vi "W7X2DPut.vi"(0 "SigLabel":string, 1 "Unit":string, 5 "SigJSONbuffer":string, 7 "values":T1(array[cluster]), 8 "dimensions":i64[](array[numeric])=[1399090569999999999, -1], 9 "sample rate":u16, 11 "sample period":dbl, 12 "pulse_length":dbl) -> (2 "headers parms":string, 3 "headers":string, 4 "body":string, 6 "body Parlog":string, 10 "file path written":string, 14 "Parlog error out":errorcluster)   [LabVIEW 2014]
uses:
  <vilib>/httpClient/POSTBuffer.vi
  <vilib>/httpClient/LabVIEWHTTPClient.lvlib
panel:
  out "JSON string":string
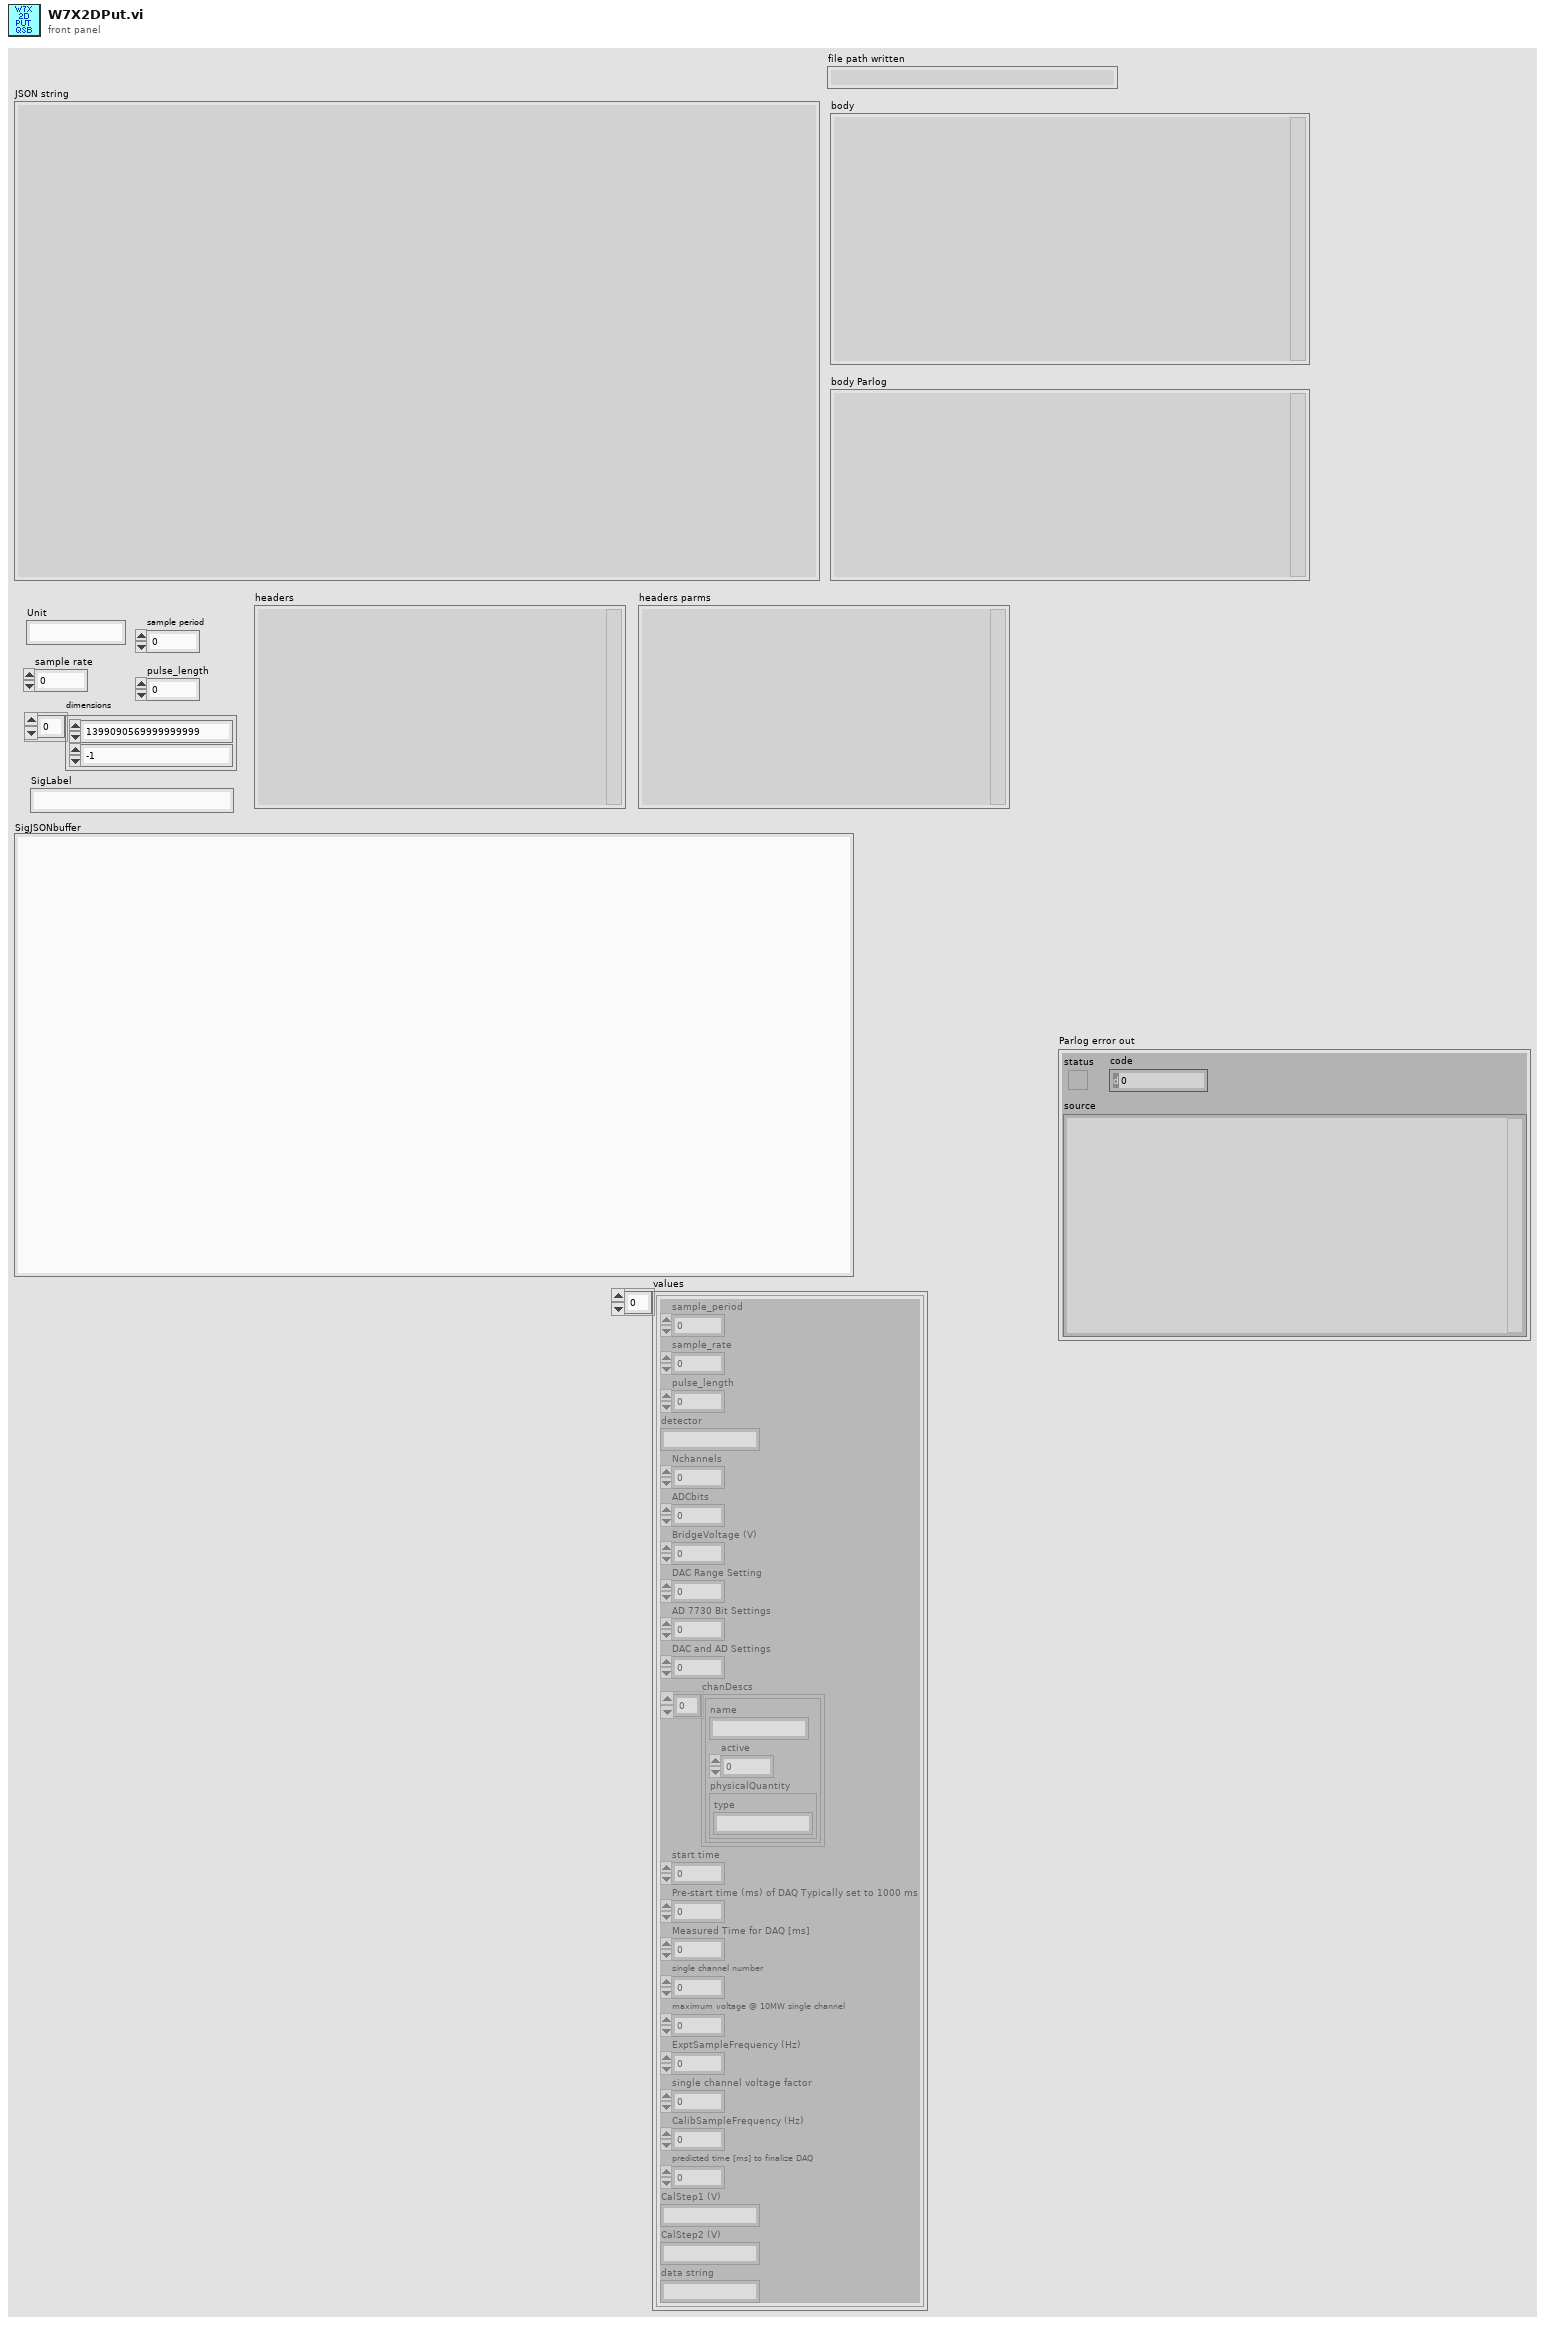
[diagram p1: front panel]
types:
  T1 = cluster{"sample_period":dbl, "sample_rate":dbl, "pulse_length":dbl, "detector":string, "Nchannels":i16, "ADCbits":i16, "BridgeVoltage (V)":sgl, "DAC Range Setting":u8, "AD 7730 Bit Settings":i32, "DAC and AD Settings":i32, "chanDescs":cluster{"name":string, "active":i32, "physicalQuantity":cluster{"type":string}}[], "start time":i64, "Pre-start time (ms) of DAQ Typically set to 1000 ms":i32, "Measured Time for DAQ [ms] ":u32, "single channel number":i64, "maximum voltage @ 10MW single channel":dbl, "ExptSampleFrequency (Hz)":sgl, "single channel voltage factor":dbl, "CalibSampleFrequency (Hz)":sgl, "predicted time [ms] to finalize DAQ":dbl, "CalStep1 (V)":string, "CalStep2 (V)":string, "data string":string}[]
  T2 = cluster{"sample_period":dbl, "sample_rate":dbl, "pulse_length":dbl, "detector":string, "Nchannels":i16, "ADCbits":i16, "BridgeVoltage (V)":sgl, "DAC Range Setting":u8, "AD 7730 Bit Settings":i32, "DAC and AD Settings":i32, "chanDescs":cluster{"name":string, "active":i32, "physicalQuantity":cluster{"type":string}}[], "start time":i64, "Pre-start time (ms) of DAQ Typically set to 1000 ms":i32, "Measured Time for DAQ [ms] ":u32, "single channel number":i64, "maximum voltage @ 10MW single channel":dbl, "ExptSampleFrequency (Hz)":sgl, "single channel voltage factor":dbl, "CalibSampleFrequency (Hz)":sgl, "predicted time [ms] to finalize DAQ":dbl, "CalStep1 (V)":string, "CalStep2 (V)":string, "data string":string}
  T3 = cluster{"name":string, "active":i32, "physicalQuantity":cluster{"type":string}}[]
  T4 = cluster{"name":string, "active":i32, "physicalQuantity":cluster{"type":string}}
  T5 = typedef "LabVIEWHTTPClient.lvlib/ClientHandle.ctl" = refnum<k1>
  T6 = cluster{"label":string, "values":cluster{"sample_period":dbl, "sample_rate":dbl, "pulse_length":dbl, "detector":string, "Nchannels":i16, "ADCbits":i16, "BridgeVoltage (V)":sgl, "DAC Range Setting":u8, "AD 7730 Bit Settings":i32, "DAC and AD Settings":i32, "chanDescs":cluster{"name":string, "active":i32, "physicalQuantity":cluster{"type":string}}[], "start time":i64, "Pre-start time (ms) of DAQ Typically set to 1000 ms":i32, "Measured Time for DAQ [ms] ":u32, "single channel number":i64, "maximum voltage @ 10MW single channel":dbl, "ExptSampleFrequency (Hz)":sgl, "single channel voltage factor":dbl, "CalibSampleFrequency (Hz)":sgl, "predicted time [ms] to finalize DAQ":dbl, "CalStep1 (V)":string, "CalStep2 (V)":string, "data string":string}[], "dimensions":i64[]}
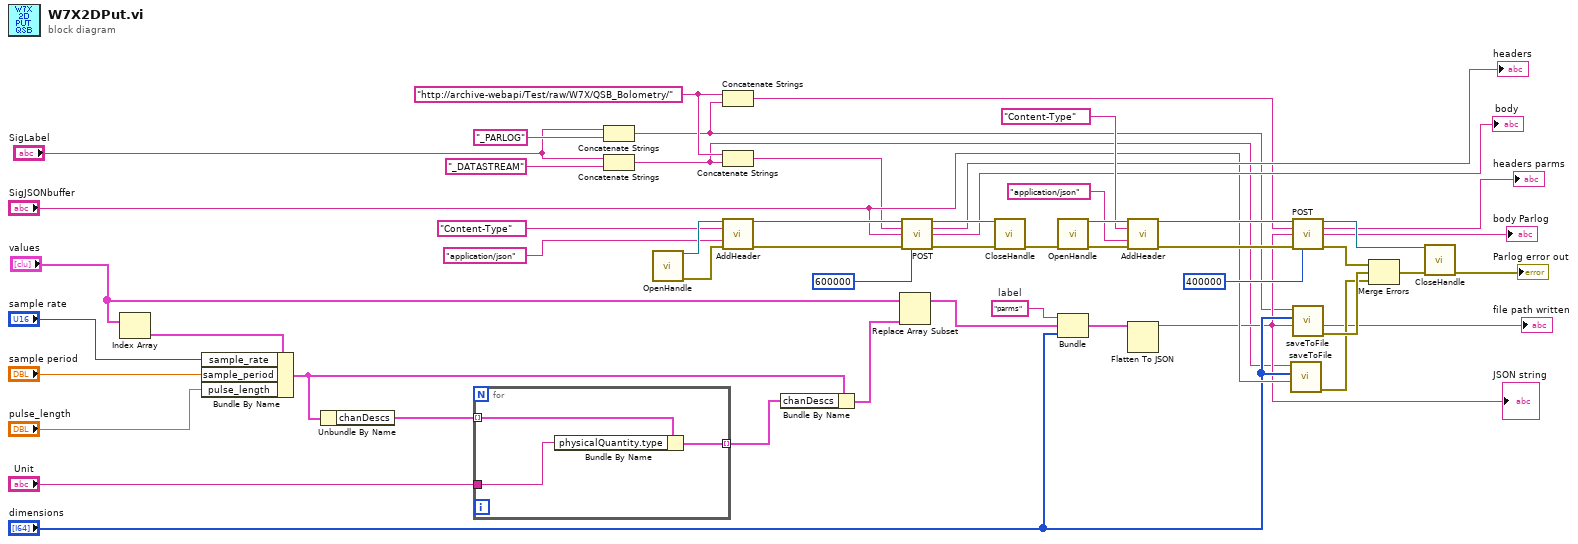
[diagram p0: block diagram]
diagram:
  w27 = "parms"  # label
  w12 = "http://archive-webapi/Test/raw/W7X/QSB_Bolometry/" ("url")
  n1 = Index Array(array="values") -> (element=w22:T2)  [unwired: 1 in]
  n2 = Bundle By Name(cluster=w22, "sample_rate"="sample rate", "sample_period"="sample period", "pulse_length"="pulse_length") -> (w19:T2)
  n3 = Unbundle By Name(w19) -> ("chanDescs"=w18:T3)
  n4 = for {
    tunnel: w18 -> [w53] mode=indexing
    tunnel: [w55] -> w17 mode=indexing
    tunnel: "Unit" -> [w54]
    n5 = Bundle By Name(cluster=w53, "physicalQuantity.type"=w54) -> (w55:T4)
  }
  n6 = Concatenate Strings("SigLabel", "_PARLOG" ("replace string (\"\")")) -> (w5:string)
  n7 = Concatenate Strings("SigLabel", "_DATASTREAM" ("string")) -> (w4:string)
  n8 = call <vilib>:"OpenHandle.vi"() -> ("client handle out"=w37:T5, "error out"=w36:errorcluster)  [unwired: 14 in]
  n9 = Concatenate Strings(w12, w5) -> (w13:string)
  n10 = Concatenate Strings(w12, w4) -> (w2:string)
  n11 = call <vilib>:"AddHeader.vi"("client handle"=w37, "header"="Content-Type", "value"="application/json", "error in (no error)"=w36) -> ("client handle out"=w35:T5, "error out"=w34:errorcluster)  [unwired: 10 in]
  n12 = Bundle By Name(cluster=w19, "chanDescs"=w17) -> (w21:T2)
  n13 = Replace Array Subset(array="values", new element=w21) -> (w20:T1)  [unwired: 1 in]
  n14 = call-poly <vilib>:"POST.vi"("client handle"=w35, "url"=w2, "buffer"="SigJSONbuffer", "error in (no error)"=w34, "timeout (10000)"=600000) -> ("client handle out"=w40:T5, "headers"=→"headers":string, "body"=→"body":string, "error out"=w39:errorcluster)  [unwired: 7 in]
  n15 = call <vilib>:"CloseHandle.vi"("client handle"=w40, "error in (no error)"=w39) -> ("error out"=w6:errorcluster)  [unwired: 13 in]
  n16 = call <vilib>:"OpenHandle.vi"("error in (no error)"=w6) -> ("client handle out"=w49:T5, "error out"=w48:errorcluster)  [unwired: 13 in]
  n17 = Bundle("label"=w27, "values"=w20, "dimensions"="dimensions") -> (w26:T6)  [unwired: 1 in]
  n18 = call <vilib>:"AddHeader.vi"("client handle"=w49, "header"="Content-Type", "value"="application/json", "error in (no error)"=w48) -> ("client handle out"=w47:T5, "error out"=w46:errorcluster)  [unwired: 10 in]
  n19 = Flatten To JSON(anything=w26) -> (JSON string=w10:string)  [unwired: 2 in, 1 out]
  "JSON string" <- w10
  n20 = call "saveToFile.vi"("SigJSONbuffer"="SigJSONbuffer", "dimensions"="dimensions", "String"=w4) -> ("error out"=w7:errorcluster)  [unwired: 7 in, 1 out]
  n21 = call-poly <vilib>:"POST.vi"("client handle"=w47, "url"=w13, "buffer"=w10, "error in (no error)"=w46, "timeout (10000)"=400000) -> ("client handle out"=w52:T5, "headers"=→"headers parms":string, "body"=→"body Parlog":string, "error out"=w51:errorcluster)  [unwired: 7 in]
  n22 = call "saveToFile.vi"("SigJSONbuffer"=w10, "dimensions"="dimensions", "String"=w5) -> ("error out"=w8:errorcluster, "resulting string"=→"file path written":string)  [unwired: 7 in]
  n23 = Merge Errors(w51, w8, w7) -> (w9:errorcluster)
  n24 = call <vilib>:"CloseHandle.vi"("client handle"=w52, "error in (no error)"=w9) -> ("error out"=→"Parlog error out":errorcluster)  [unwired: 13 in]
